vi "NIIE_Global Data.vi"() -> ()   [LabVIEW 2021]
uses:
  vi.lib/LabVIEW Icon API/lv_icon/Controls/IEColor.ctl
panel:
  in  "All Glyphs":string="All Glyphs"
  in  "All Templates":string="All Templates"
  in  "Layer Color":T1=16762457
  in  "Template Color":T1=12303291
  in  "Layer Clust":T2={"Minimum # of selected elements"=1, "Maximum # of selected elements"=1, "# Rows"=4, "# Cols"=1}
  in  "Framework Templates":T2={"Minimum # of selected elements"=0, "Maximum # of selected elements"=1, "# Rows"=5, "# Cols"=6}
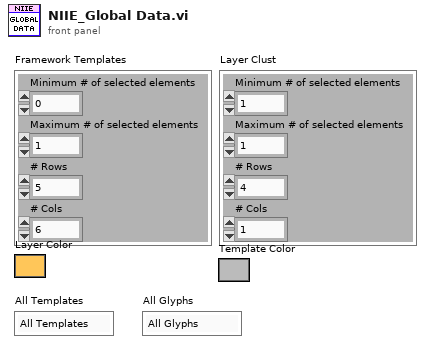
[diagram p1: front panel]
types:
  T1 = typedef "IEColor.ctl" = u32
  T2 = cluster{"Minimum # of selected elements":u32, "Maximum # of selected elements":u32, "# Rows":u32, "# Cols":u32}
diagram:
